vi "SrvSetCpuStatus.vi"(0 "ref in":u64, 7 "CpuStatus":i32(ring)=8 items=["Run"=8, "Stop"=4], 11 "error in (no error)":errorcluster) -> (4 "ref out":u64, 8 "return type":i32, 15 "error out":errorcluster)   [LabVIEW 2016, in "Snap7.lvlib"]
uses:
  Snap7.lvlib
  win32/lv_snap7.dll
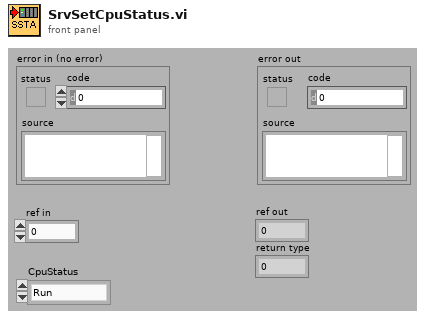
[diagram p1: front panel]
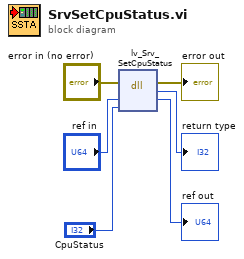
[diagram p0: block diagram]
diagram:
  n1 = dll-call lib="D:/maszup/svn/LineTraceSystem/SOFTWARE/sources/Drivers/PLC/Snap7/lib/win32/lv_snap7.dll" fn="lv_Srv_SetCpuStatus"(error in="error in (no error)", "Server"="ref in", "Status"="CpuStatus") -> (error out=→"error out":errorcluster, "return type"=→"return type":i32, "Server"=→"ref out":u64)  [unwired: 3 in, 1 out]
